vi "BattlesonEXCt2.VI.vi"() -> ()   [LabVIEW 2014, in "Battleson_Robot_12-2-16.lvrbt"]
uses:
  C:/Users/blb1094/Documents/LabVIEW Data/NXTRobotics/Projects/Battleson_Robot_12-2-16/Battleson_Robot_12-2-16.lvrbt
  <vilib>/NXT/Block Support/NXT_InputPort.ctl
  <vilib>/NXT/Block Support/NXT_OutputPort.ctl
  <vilib>/NXT/Dual Mode Library/Sensors/EV3_Ultrasonic_CM.vi
  <vilib>/NXT/NXTIO Xnodes/NXTIONodeSubVIs/NXTMoveMotors.vi
  <vilib>/NXT/Subs/LVHSConnector.ctl
  <vilib>/NXT/NXTIO Xnodes/AddressXNode/NXTIOAddress.xnode
  <vilib>/NXT/NXTIO Xnodes/NXTIOXNode/NXTIO.xnode
  <vilib>/NXT/LegoClasses/BrickReference/BrickReference.lvclass
panel:
  in  "stop":bool
  out "Distance From Wall":dbl
  out "Number of Loop iterations":i32
  out "Final Iteration":i32
  out "current iteration":i32
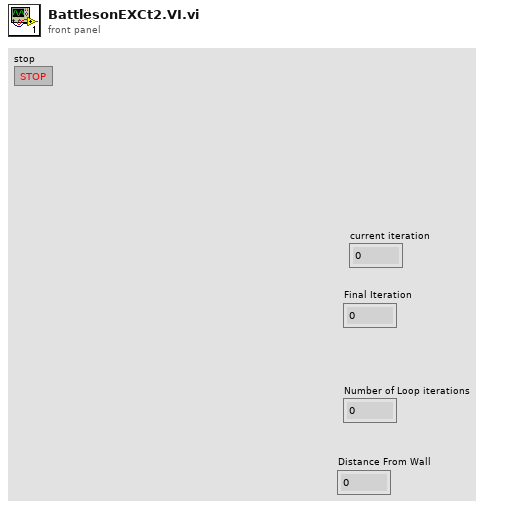
[diagram p1: front panel]
types:
  T1 = typedef "NXT_OutputPort.ctl" = u8
  T2 = typedef "NXT_InputPort.ctl" = u32
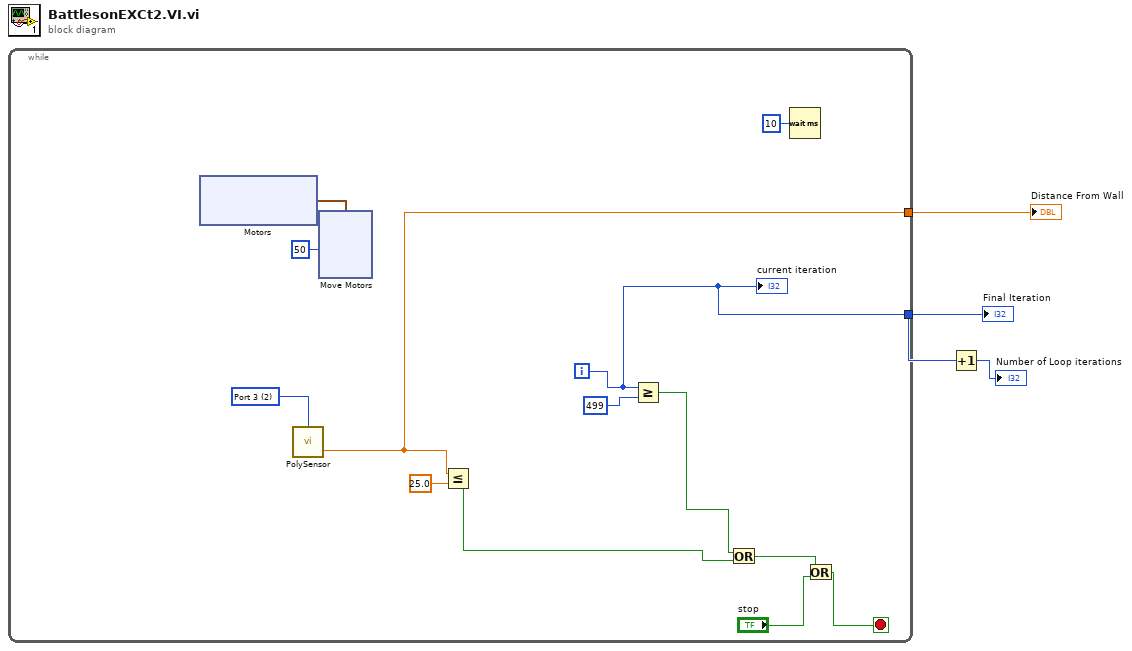
[diagram p0: block diagram]
diagram:
  n1 = while {
    tunnel: [w5] -> w1
    tunnel: [w4] -> w3
    i -> [w5]
    stop <- w12 stop-if-true
    w13 = i8 50 ("Power/Speed 1")
    w15 = T2 2 items=["Port 1", "Port 2", "Port 3", "Port 4"] ("Port (Port 1)")
    n2 = xnode "Motors"() -> ("Motor"=w14:cluster{"Port":T1, "Port":T1})
    n3 = call-poly <vilib>:"PolySensor.vi"("Port (Port 1)"=w15) -> ("Centimeters"=w4:sgl)  [unwired: 2 in, 1 out]
    n4 = xnode "Move Motors"("Power/Speed 2"=w13, "Power/Speed 1"=w13, "Motors"=w14) -> ()  [unwired: 1 in, 1 out]
    n5 = Less Or Equal?(x=w4, y=25.0) -> (x <= y?=w9:bool)
    n6 = Greater Or Equal?(x=w5, y=499) -> (x >= y?=w7:bool)
    n7 = Or(x=w7, y=w9) -> (x .or. y?=w10:bool)
    n8 = Wait (ms)(milliseconds to wait=u32 10) -> ()  [unwired: 1 out]
    n9 = Or(x=w10, y="stop") -> (x .or. y?=w12:bool)
    "current iteration" <- w5
  }
  "Final Iteration" <- w1
  "Distance From Wall" <- w3
  n10 = Increment(x=w1) -> (x+1=→"Number of Loop iterations":i32)
